vi "AOL Z Cal-Fine-tuning algorithm.vi"(8 "error in (no error)":errorcluster, 9 "Max offset (us)":i32=30 min=5 max=100, 10 "Wait before measurement (ms)":u32=200, 11 "Initial motor position (um)":sgl) -> (0 "error out":errorcluster, 3 "Measured cal value":sgl)   [LabVIEW 2013]
panel:
  out "Motor pos of max intensity during upwards movement":sgl
  out "Motor pos of max intensity  during downwards movement":sgl
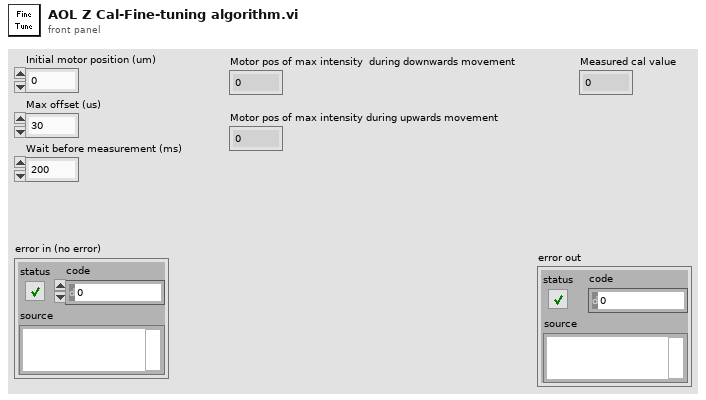
[diagram p1: front panel]
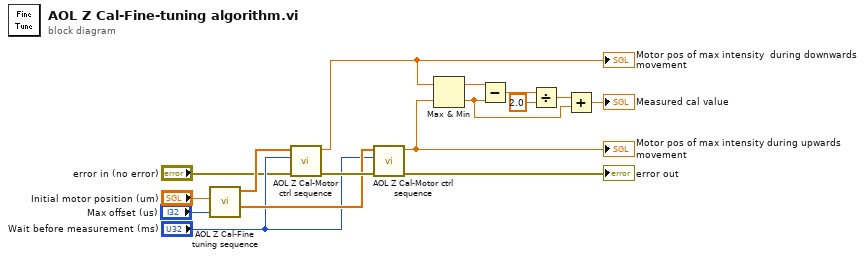
[diagram p0: block diagram]
diagram:
  n1 = call "AOL Z Cal-Fine tuning sequence.vi"("Max offset (us)"="Max offset (us)", "Initial value"="Initial motor position (um)") -> ("Ascending sequence"=w12:sgl[], "Descending sequence"=w15:sgl[])  [unwired: 8 in]
  n2 = call "AOL Z Cal-Motor ctrl sequence.vi"("error in (no error)"="error in (no error)", "Wait before measurement (ms)"="Wait before measurement (ms)", "Motor positions sequence"=w15) -> ("error out"=w14:errorcluster, "Motor pos at max intensity"=w3:sgl)  [unwired: 7 in]
  "Motor pos of max intensity  during downwards movement" <- w3
  n3 = call "AOL Z Cal-Motor ctrl sequence.vi"("error in (no error)"=w14, "Wait before measurement (ms)"="Wait before measurement (ms)", "Motor positions sequence"=w12) -> ("error out"=→"error out":errorcluster, "Motor pos at max intensity"=w10:sgl)  [unwired: 7 in]
  "Motor pos of max intensity during upwards movement" <- w10
  n4 = Max & Min(x=w3, y=w10) -> (max(x,y)=w9:sgl, min(x,y)=w5:sgl)
  n5 = Subtract(x=w9, y=w5) -> (x-y=w8:sgl)
  n6 = Divide(x=w8, y=sgl 2.0) -> (x/y=w6:sgl)
  n7 = Add(x=w6, y=w5) -> (x+y=→"Measured cal value":sgl)
